vi "Send Self-Addressed Message.vi"(8 "error in (no error)":errorcluster, 11 "Self-Addressed Message in":refnum<class "Self-Addressed Msg.lvclass">) -> (0 "error out":errorcluster, 3 "Self-Addressed Message out":refnum<class "Self-Addressed Msg.lvclass">)   [LabVIEW 2017, in "AF_Messages-PPL.lvlib" / "Self-Addressed Msg.lvclass"]
doc: "(<B>Filename</B>: Actor Framework.lvlib:Self-Addressed Msg.lvclass:Send Self-Addressed Message.vi)\n\nSends a self-addressed message. You can send multiple copies to the same address by calling this VI multiple times with the same message.\n\nUse the Address Message method to create a self-addressed message."
uses:
  Self-Addressed Msg.lvclass
  Self-Addressed Msg.lvclass/Self-Addressed Msg.ctl
  Actor Framework.lvlibp/1abvi3w/vi.lib/ActorFramework/Message Enqueuer/Message Enqueuer.lvclass
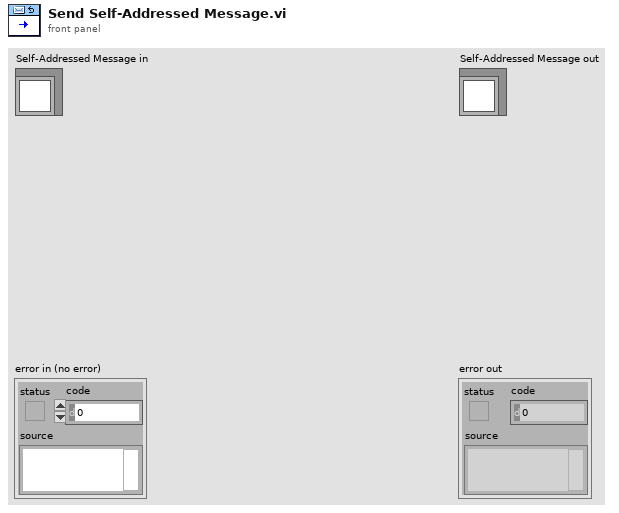
[diagram p1: front panel]
types:
  T1 = typedef "Actor Framework.lvlibp/Message Enqueuer.lvclass/Message Priority.ctl" = enum16{"Low", "Normal", "High"}
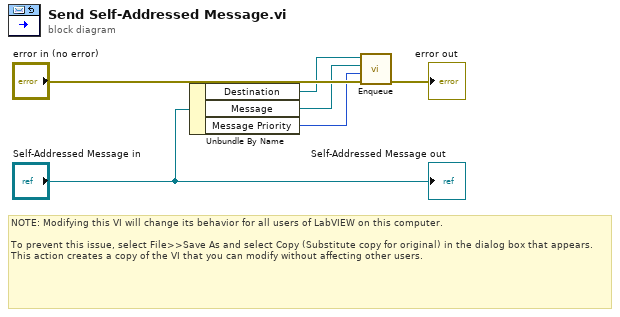
[diagram p0: block diagram]
diagram:
  # "NOTE: Modifying this VI will change its behavior for all users of LabVIEW on this computer.\n\nTo prevent this issue, select File>>Save As and select Copy (Substitute copy for original) in the dialog box that appears. This action creates a copy of the VI that you can modify without affecting other users."
  n1 = Unbundle By Name("Self-Addressed Message in") -> ("Destination"=w3:refnum<class "Message Enqueuer.lvclass">, "Message"=w2:refnum<class "Message.lvclass">, "Message Priority"=w1:T1)
  n2 = call "Enqueue.vi"("error in (no error)"="error in (no error)", "Message Priority (Normal)"=w1, "Message"=w2, "Message Enqueuer in"=w3) -> ("error out"=→"error out":errorcluster)  [unwired: 6 in, 1 out]
  "Self-Addressed Message out" <- "Self-Addressed Message in"
